vi "SetupFile_GetElapsedDuration.vi"(11 "Path":path) -> (3 "date/time string":string)   [LabVIEW 2024]
uses:
  <vilib>/Utility/file.llb/Read Delimited Spreadsheet (string).vi
panel:
  out "error out 2":errorcluster
  out "error out":errorcluster
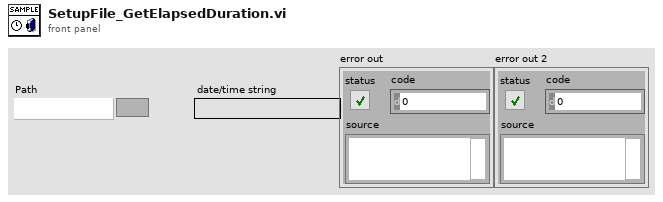
[diagram p1: front panel]
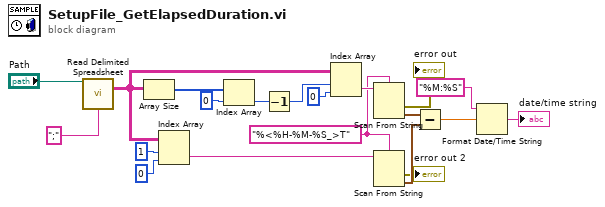
[diagram p0: block diagram]
diagram:
  w14 = "%<%H-%M-%S_>T" ("time format string (%c)")
  n1 = call-poly <vilib>:"Read Delimited Spreadsheet.vi"("file path (dialog if empty)"="Path", "delimiter (\\t)"=";" ("delimiter (\\t)")) -> ("all rows"=w9:string[][])  [unwired: 8 in, 5 out]
  n2 = Array Size(array=w9) -> (size(s)=w10:i32[])
  n3 = Index Array(array=w9, index (row)=1, index (col)=0 ("disabled index (col)")) -> (element=w13:string)
  n4 = Index Array(array=w10, index=0) -> (element=w12:i32)
  n5 = Decrement(x=w12) -> (x-1=w3:i32)
  n6 = Index Array(array=w9, index (row)=w3, index (col)=0 ("disabled index (col)")) -> (element=w15:string)
  n7 = Scan From String(format string=w14, input string=w15) -> (error out=→"error out":errorcluster, output 1=w16:timestamp)  [unwired: 3 in, 2 out]
  n8 = Scan From String(format string=w14, input string=w13) -> (error out=→"error out 2":errorcluster, output 1=w17:timestamp)  [unwired: 3 in, 2 out]
  n9 = Subtract(x=w16, y=w17) -> (x-y=w19:dbl)
  n10 = Format Date/Time String(time format string (%c)="%M:%S", seconds (now)=w19) -> (date/time string=→"date/time string":string)  [unwired: 1 in]
